vi "looking at waterr140.vi"() -> ()   [LabVIEW 2020]
uses:
  common/record_file_handler/VFH-file_cluster-r140.ctl
  common/record_file_handler/VFH-VNA_File_Handler.lvlib
panel:
  in  "Water Temp":dbl=28.0 format="%#_13g"
  out "Handled data":T1
  out "Raw 2":cluster{"Frequency":dbl[], "S21_Imag":dbl[]}[](graph)
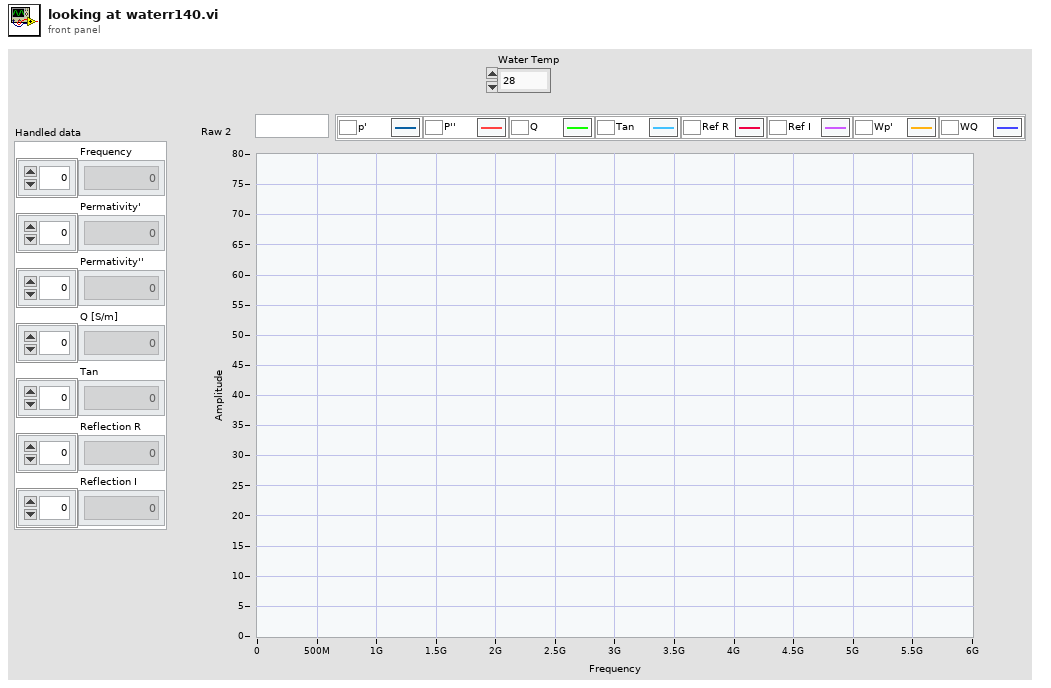
[diagram p1: front panel]
types:
  T1 = typedef "VFH-VNA_File_Handler.lvlib/VFH-file_cluster-r140.ctl" = cluster{"Frequency":dbl[], "Permativity'":dbl[], "Permativity''":dbl[], "Q [S/m]":dbl[], "Tan":dbl[], "Reflection R":dbl[], "Reflection I":dbl[]}
  T2 = typedef "VFH-VNA_File_Handler.lvlib/VFH-file_cluster-r140_water.ctl" = cluster{"Frequency":dbl[], "Permativity'":dbl[], "Q [S/m]":dbl[]}
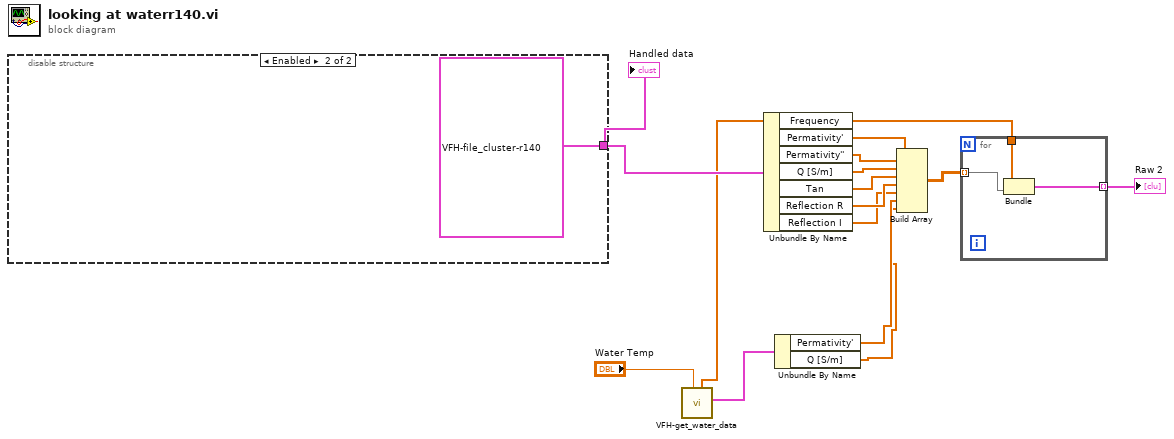
[diagram p0: block diagram]
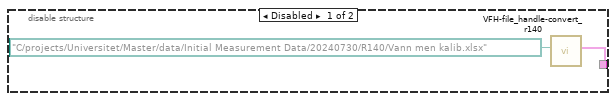
[diagram p2: hidden frame]
diagram:
  n1 = disable-structure shown="Enabled" {
    disable-tunnel: [w15 T1 {"Frequency"=[300000000.0, 350000000.0, 400000000.0, 450000000.0, 500000000.0, 550000000.0, 600000000.0, 650000000.0, 700000000.0, 750000000.0, 800000000.0, 850000000.0, 900000000.0, 950000000.0, 1000000000.0, 1050000000.0, 1100000000.0, 1150000000.0, 1200000000.0, 1250000000.0, 1300000000.0, 1350000000.0, 1400000000.0, 1450000000.0, 1500000000.0, 1550000000.0, 1600000000.0, 1650000000.0, 1700000000.0, 1750000000.0, 1800000000.0, 1850000000.0, 1900000000.0, 1950000000.0, 2000000000.0, 2050000000.0, 2100000000.0, 2150000000.0, 2200000000.0, 2250000000.0, 2300000000.0, 2350000000.0, 2400000000.0, 2450000000.0, 2500000000.0, 2550000000.0, 2600000000.0, 2650000000.0, 2700000000.0, 2750000000.0, 2800000000.0, 2850000000.0, 2900000000.0, 2950000000.0, 3000000000.0, 3050000000.0, 3100000000.0, 3150000000.0, 3200000000.0, 3250000000.0, 3300000000.0, 3350000000.0, 3400000000.0, 3450000000.0, 3500000000.0, 3550000000.0, 3600000000.0, 3650000000.0, 3700000000.0, 3750000000.0, 3800000000.0, 3850000000.0, 3900000000.0, 3950000000.0, 4000000000.0, 4050000000.0, 4100000000.0, 4150000000.0, 4200000000.0, 4250000000.0, 4300000000.0, 4350000000.0, 4400000000.0, 4450000000.0, 4500000000.0, 4550000000.0, 4600000000.0, 4650000000.0, 4700000000.0, 4750000000.0, 4800000000.0, 4850000000.0, 4900000000.0, 4950000000.0, 5000000000.0, 5050000000.0, 5100000000.0, 5150000000.0, 5200000000.0, 5250000000.0, 5300000000.0, 5350000000.0, 5400000000.0, 5450000000.0, 5500000000.0, 5550000000.0, 5600000000.0, 5650000000.0, 5700000000.0, 5750000000.0, 5800000000.0, 5850000000.0, 5900000000.0, 5950000000.0], "Permativity'"=[79.43406000000002, 79.43674, 79.433, 79.42808, 79.42496, 79.41688, 79.41004000000001, 79.39796, 79.3835, 79.37044, 79.35528, 79.33462, 79.31604, 79.29440000000001, 79.27448, 79.26097999999999, 79.24542, 79.22510000000001, 79.20439999999999, 79.1835, 79.1618, 79.1439, 79.12192, 79.09559999999999, 79.06801999999999, 79.0367, 79.00138, 78.96606, 78.92715999999999, 78.88398, 78.83818, 78.78972, 78.73537999999999, 78.67620000000001, 78.62606000000001, 78.57808000000001, 78.53554, 78.49104, 78.4477, 78.40542, 78.36268, 78.32154, 78.27941999999999, 78.23375999999999, 78.18472, 78.12904, 78.06392, 77.98743999999999, 77.90272000000002, 77.81334000000001, 77.72313999999999, 77.63374000000002, 77.54576, 77.46119999999999, 77.37805999999999, 77.29534000000001, 77.21387999999999, 77.13466000000001, 77.05427999999999, 76.97754, 76.904, 76.83416000000001, 76.76483999999999, 76.68796, 76.61422, 76.53678000000001, 76.45478, 76.36746, 76.28098, 76.19618, 76.11466, 76.03432, 75.9515, 75.86228000000001, 75.76494, 75.66299999999998, 75.56861999999998, 75.48177999999999, 75.37078, 75.25537999999999, 75.15486000000001, 75.06008, 74.97008, 74.88828, 74.80668, 74.73173999999999, 74.63918, 74.57075999999999, 74.49256, 74.41688, 74.34486000000001, 74.2788, 74.21853999999999, 74.15788, 74.0898, 74.00796, 73.9256, 73.82458, 73.73373999999998, 73.64957999999999, 73.57136, 73.49506, 73.40617999999999, 73.32667999999998, 73.23954, 73.15588, 73.08008, 72.99629999999999, 72.87533999999998, 72.75046, 72.62983999999999, 72.499, 72.38247999999999, 72.24182], "Permativity''"=[1.4254640000000003, 1.6989740000000002, 1.9193380000000002, 2.1000199999999998, 2.2711999999999994, 2.446312, 2.624868, 2.813602, 3.0064279999999997, 3.208658, 3.4140699999999997, 3.6219360000000003, 3.8288939999999996, 4.032870000000001, 4.235722, 4.437676, 4.641912, 4.846676, 5.051302, 5.252708, 5.454426, 5.656672, 5.861458000000001, 6.0651399999999995, 6.2710799999999995, 6.476072, 6.682267999999999, 6.88865, 7.097148, 7.302930000000001, 7.506944, 7.70732, 7.904218, 8.092229999999999, 8.283555999999999, 8.476172, 8.671402, 8.867892, 9.065050000000001, 9.266156, 9.470138, 9.677912, 9.889262, 10.09972, 10.3101, 10.516359999999999, 10.72148, 10.92782, 11.134960000000001, 11.33982, 11.5448, 11.747, 11.94414, 12.131959999999998, 12.31208, 12.48776, 12.66374, 12.844220000000002, 13.03016, 13.218859999999998, 13.40758, 13.59546, 13.77998, 13.95838, 14.138919999999999, 14.320060000000002, 14.50676, 14.69544, 14.883139999999997, 15.074360000000002, 15.26248, 15.44638, 15.625, 15.79844, 15.9695, 16.13724, 16.307760000000002, 16.48344, 16.659699999999997, 16.83612, 17.005280000000003, 17.17364, 17.33348, 17.49452, 17.64938, 17.81218, 17.97654, 18.152579999999997, 18.32064, 18.487920000000003, 18.65864, 18.82464, 18.980020000000003, 19.11994, 19.283160000000002, 19.4352, 19.583500000000004, 19.749239999999997, 19.919919999999998, 20.0948, 20.264780000000002, 20.42666, 20.583180000000002, 20.721119999999996, 20.859019999999997, 21.01946, 21.17048, 21.33104, 21.50074, 21.6766, 21.842999999999996, 22.003719999999998, 22.16498, 22.321400000000004], "Q [S/m]"=[0.02379012, 0.03308064, 0.042710139999999994, 0.0525721, 0.06317496, 0.07485032, 0.08761494, 0.1017408, 0.1170762, 0.13387640000000003, 0.151943, 0.17126899999999998, 0.1917056, 0.21313620000000003, 0.23563900000000002, 0.2592174, 0.2840592, 0.3100708, 0.3372128, 0.36526859999999994, 0.394468, 0.4248291999999999, 0.45651260000000005, 0.4892472, 0.5233025999999998, 0.5584224, 0.5947896, 0.6323208, 0.6712005999999999, 0.7109754, 0.7517178000000001, 0.7932218000000001, 0.8354718, 0.8778539999999999, 0.9216504000000001, 0.9666584, 1.013044, 1.0606659999999999, 1.1094620000000002, 1.15985, 1.211722, 1.26523, 1.3203679999999998, 1.376558, 1.433914, 1.4918479999999998, 1.550772, 1.611012, 1.672524, 1.734834, 1.798308, 1.8624800000000001, 1.92696, 1.9910039999999998, 2.054808, 2.1188659999999997, 2.183954, 2.2508, 2.319632, 2.389996, 2.461408, 2.533716, 2.606436, 2.679004, 2.7529820000000003, 2.828086, 2.9053080000000002, 2.983966, 3.063482, 3.144768, 3.22647, 3.308318, 3.3900419999999998, 3.4716099999999996, 3.553622, 3.635828, 3.719612, 3.8055320000000004, 3.892564, 3.9806179999999998, 4.067916, 4.155954, 4.242849999999999, 4.33093, 4.418362, 4.508658, 4.600274000000001, 4.6958079999999995, 4.790252000000001, 4.88541, 4.98242, 5.079114, 5.173828, 5.265152, 5.36374, 5.460088000000001, 5.556236, 5.658186, 5.76249, 5.868974, 5.97499, 6.079532, 6.183376, 6.2824539999999995, 6.382276, 6.489848, 6.595354, 6.70471, 6.817854, 6.933912000000001, 7.047896, 7.160953999999999, 7.2751019999999995, 7.388536], "Tan"=[0.01794524, 0.02138774, 0.02416298, 0.02643928, 0.028595560000000003, 0.030803399999999998, 0.03305462, 0.0354367, 0.03787224, 0.04042636, 0.04302258, 0.045653900000000004, 0.048273899999999995, 0.0508595, 0.053431099999999995, 0.05598814, 0.05857642, 0.06117598, 0.06377552, 0.0663359, 0.06890226, 0.07147322, 0.07408132, 0.07668114000000001, 0.07931246, 0.08193754, 0.08458418000000001, 0.0872356, 0.08992022000000002, 0.09257814, 0.09521958, 0.09782142, 0.1003896, 0.1028548, 0.10535380000000001, 0.1078694, 0.1104138, 0.1129796, 0.1155554, 0.11818279999999999, 0.12084999999999999, 0.1235664, 0.12633280000000002, 0.1290966, 0.1318686, 0.1346024, 0.1373424, 0.1401226, 0.1429344, 0.14573080000000002, 0.1485376, 0.15131319999999998, 0.15402719999999998, 0.1566198, 0.15911560000000002, 0.16155880000000003, 0.16400900000000002, 0.16651639999999998, 0.169104, 0.1717238, 0.17434180000000002, 0.1769456, 0.179509, 0.1820154, 0.18454700000000002, 0.18710020000000002, 0.189743, 0.1924306, 0.1951094, 0.19783599999999998, 0.20051979999999997, 0.2031502, 0.20572340000000003, 0.2082516, 0.210777, 0.2132774, 0.21580080000000001, 0.21837660000000003, 0.2210366, 0.22371999999999997, 0.22626999999999997, 0.2287982, 0.2312052, 0.23360820000000002, 0.2359332, 0.23834820000000004, 0.2408462, 0.24342740000000002, 0.24593959999999998, 0.2484372, 0.25097420000000004, 0.2534324, 0.2557312, 0.2578274, 0.26026760000000004, 0.2626096, 0.2649086, 0.2675162, 0.2701602, 0.2728434, 0.27544399999999997, 0.2779322, 0.2804014, 0.2825866, 0.28480540000000004, 0.2873248, 0.28968859999999996, 0.2922212, 0.2950348, 0.2979584, 0.3007442, 0.3035036, 0.3062204, 0.3089822], "Reflection R"=[0.9566874000000001, 0.941441, 0.9245432000000001, 0.9055994, 0.8850052000000002, 0.8627768, 0.8388036, 0.8132962000000001, 0.7869998, 0.759286, 0.7308222, 0.7015254000000001, 0.6717172, 0.6408704000000001, 0.6100459999999999, 0.5785362000000001, 0.5465755999999999, 0.5150712000000001, 0.48419439999999997, 0.4523198, 0.4211922, 0.3898626, 0.3592016, 0.3289972, 0.2989214, 0.26938340000000005, 0.2405052, 0.2120692, 0.1849584, 0.1578932, 0.1309398, 0.1052516, 0.0802934, 0.056137080000000006, 0.03276710000000001, 0.009347254000000001, -0.01330974, -0.03511446, -0.05617168, -0.07671984, -0.09669028, -0.11615660000000001, -0.1353046, -0.1536204, -0.17114359999999998, -0.18812540000000003, -0.2045134, -0.22041400000000003, -0.23406120000000002, -0.248726, -0.2630972, -0.27700420000000003, -0.2900322, -0.30242900000000006, -0.3142702, -0.325867, -0.3375228, -0.3488098, -0.35999780000000003, -0.37066720000000003, -0.3809134, -0.39126199999999994, -0.4005642, -0.40931280000000003, -0.41772259999999994, -0.425751, -0.4337606, -0.44163800000000003, -0.44978759999999995, -0.45763039999999994, -0.465216, -0.472266, -0.4788604, -0.4845738, -0.4904992, -0.4963558, -0.502328, -0.5084565999999999, -0.5142338000000001, -0.5196301999999999, -0.5247008, -0.5291382, -0.5332779999999999, -0.5379756, -0.5425076000000001, -0.547444, -0.552264, -0.5570352, -0.5611584, -0.5646566, -0.5679128, -0.572214, -0.5778909999999999, -0.579572, -0.5817140000000001, -0.5860828, -0.5893008, -0.5926888, -0.5959652, -0.5990956000000001, -0.6025456, -0.603111, -0.6074686, -0.6097471999999999, -0.6120062, -0.6136482000000001, -0.6155649999999999, -0.6181858, -0.6217192, -0.6231867999999999, -0.6252142, -0.6287453999999999, -0.6286804, -0.6303856000000001], "Reflection I"=[-0.2738478, -0.3169812, -0.358823, -0.3994014, -0.4387966, -0.47618779999999994, -0.51262, -0.5471293999999999, -0.579743, -0.6106992, -0.6400734000000001, -0.6673206, -0.6932546, -0.7170378000000001, -0.7391132, -0.7596011999999999, -0.7785314000000001, -0.7948294, -0.8106132, -0.8246492, -0.8368211999999999, -0.8479628, -0.8571696, -0.8654836000000001, -0.8723116, -0.877876, -0.8823013999999999, -0.8856683999999999, -0.8883230000000001, -0.889898, -0.8909914000000001, -0.8907453999999999, -0.8895298, -0.8877656, -0.8858372000000001, -0.8830772, -0.8798486000000001, -0.8759966, -0.8720890000000001, -0.8675386000000002, -0.8624930000000001, -0.8570008, -0.851123, -0.8447578, -0.8383524000000001, -0.8312302, -0.8241642, -0.8170162, -0.8108166000000001, -0.803769, -0.7962894, -0.7886371999999999, -0.7813450000000001, -0.7742826, -0.7672030000000001, -0.7597683999999999, -0.7520937999999999, -0.7441241999999999, -0.7363958, -0.7287334, -0.7214154, -0.7142196000000001, -0.7069799999999999, -0.6996656, -0.6925606, -0.6847032, -0.6767994, -0.6689806, -0.6615832, -0.6547532, -0.6477106, -0.6408988, -0.6339319999999999, -0.6270486, -0.6200452000000001, -0.6129746, -0.6057774, -0.598859, -0.5927054, -0.5865866000000001, -0.5805484, -0.5742032, -0.567995, -0.5618434000000001, -0.5550454, -0.548258, -0.5418732, -0.5359619999999999, -0.5305096, -0.5253042, -0.5200322, -0.513817, -0.5065594000000001, -0.5014108, -0.49582560000000003, -0.4899918, -0.48413680000000003, -0.4793794, -0.473677, -0.46922239999999993, -0.46334279999999994, -0.4595546, -0.4524427999999999, -0.44837979999999994, -0.44384239999999997, -0.43819379999999997, -0.4330426, -0.4282718, -0.424643, -0.41798959999999996, -0.4143324, -0.41060040000000003, -0.4063578, -0.4017794]} ("Handled data")] -> w6
    frame Disabled {
      n2 = call "VFH-file_handle-convert_r140.vi"("file path (dialog if empty)"=path "C:/projects/Universitet/Master/data/Initial Measurement Data/20240730/R140/Vann men kalib.xlsx") -> ("Handled data"=w15:T1)  [unwired: 10 in]
    }
    frame Enabled {
    }
  }
  "Handled data" <- w6
  n3 = Unbundle By Name(w6) -> ("Frequency"=w5:dbl[], "Permativity'"=w14:dbl[], "Permativity''"=w13:dbl[], "Q [S/m]"=w12:dbl[], "Tan"=w11:dbl[], "Reflection R"=w8:dbl[], "Reflection I"=w7:dbl[])
  n4 = call "VFH-get_water_data.vi"("Xi"=w5, "Water Temp"="Water Temp") -> ("Water Cluster"=w3:T2)  [unwired: 9 in]
  n5 = Unbundle By Name(w3) -> ("Permativity'"=w2:dbl[], "Q [S/m]"=w1:dbl[])
  n6 = Build Array(w14, w13, w12, w11, w8, w7, w2, w1) -> (w10:dbl[][])
  n7 = for {
    tunnel: w10 -> [w20] mode=indexing
    tunnel: [w19] -> w9 mode=indexing
    tunnel: w5 -> [w18]
    n8 = Bundle("Frequency"=w18, w20) -> (w19:cluster{"Frequency":dbl[], dbl[]})  [unwired: 1 in]
  }
  "Raw 2" <- w9
